vi "destroy function.vi"(11 "command in":string[](array[string])) -> ()   [LabVIEW 2011]
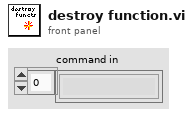
[diagram p1: front panel]
types:
  T1 = typedef "WPI_MotorControlDeviceRef.ctl" = cluster{"DeviceStatus":errorcluster, "Type":enum16{"PWM", "CAN"}, "PWM":cluster{"Digital Module":T2, "PWM Channel":T3, "DeadBand":T4}, "CAN":cluster{"Device Number":u8, "Control Mode":T5, "Semaphore":T6, "Max Vout":dbl}, "Invert":bool, "TransformRef":T7, "InvTransformRef":T7}
  T2 = typedef "FPGA_TypedefDigitalModule.ctl" = enum16{"Digital Module 1", "Digital Module 2"}
  T3 = typedef "FPGA_DIOPWMChannel.ctl" = enum8{"PWM 1", "PWM 2", "PWM 3", "PWM 4", "PWM 5", "PWM 6", "PWM 7", "PWM 8", "PWM 9", "PWM 10", "Invalid"}
  T4 = typedef "WPI_PWMDeadband.ctl" = cluster{"Name":string, "maxPositivePwm":i32, "minPositivePwm":i32, "centerPwm":i32, "maxNegativePwm":i32, "minNegativePwm":i32, "angularRange":u16}
  T5 = typedef "WPI_CANJaguar_ControlMode.ctl" = enum8{"Percent VBus", "Current", "Speed", "Position", "Voltage"}
  T6 = typedef "Semaphore RefNum" = refnum<k1>
  T7 = typedef "WPI_PWMTransform_ConPane.ctl" = refnum<vi>
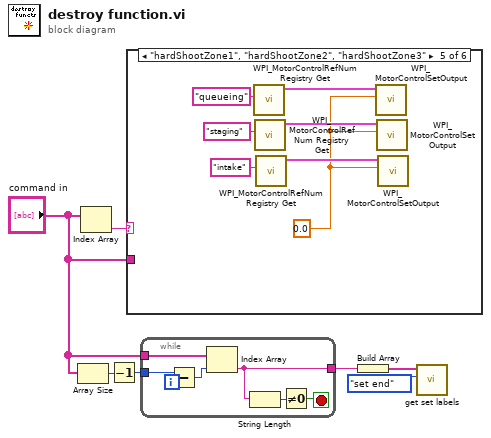
[diagram p0: block diagram]
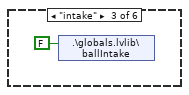
[diagram p4: hidden frame]
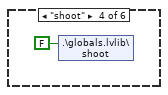
[diagram p5: hidden frame]
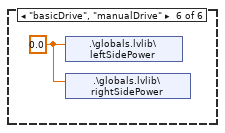
[diagram p6: hidden frame]
diagram:
  n1 = Array Size(array="command in") -> (size(s)=w6:i32)
  n2 = Index Array(array="command in") -> (element=w7:string)  [unwired: 1 in]
  n3 = Decrement(x=w6) -> (x-1=w5:i32)
  n4 = case shown="\"hardShootZone1\", \"hardShootZone2\", \"hardShootZone3\"" w7 {
    tunnel: "command in" -> [_ _ _ _ _ _]
    frame "testFunct" {
    }
    frame Default {
    }
    frame "intake" {
      n5 = shared-variable ".\\globals.lvlib\\ballIntake"(FALSE ("ballIntake")) -> ()  [unwired: 1 in, 1 out]
    }
    frame "shoot" {
      n6 = shared-variable ".\\globals.lvlib\\shoot"(FALSE ("shoot")) -> ()  [unwired: 1 in, 1 out]
    }
    frame "hardShootZone1", "hardShootZone2", "hardShootZone3" {
      w10 = 0.0 ("Output")
      n7 = call <vilib>:"WPI_MotorControlRefNum Registry Get.vi"("refnum name"="queueing") -> ("MotorControlDevRef"=w15:T1)  [unwired: 9 in, 1 out]
      n8 = call <vilib>:"WPI_MotorControlRefNum Registry Get.vi"("refnum name"="staging") -> ("MotorControlDevRef"=w14:T1)  [unwired: 9 in, 1 out]
      n9 = call <vilib>:"WPI_MotorControlRefNum Registry Get.vi"("refnum name"="intake") -> ("MotorControlDevRef"=w13:T1)  [unwired: 9 in, 1 out]
      n10 = call <vilib>:"WPI_MotorControlSetOutput.vi"("Output"=w10, "MotorControlDevRef"=w15) -> ()  [unwired: 8 in, 2 out]
      n11 = call <vilib>:"WPI_MotorControlSetOutput.vi"("Output"=w10, "MotorControlDevRef"=w14) -> ()  [unwired: 8 in, 2 out]
      n12 = call <vilib>:"WPI_MotorControlSetOutput.vi"("Output"=w10, "MotorControlDevRef"=w13) -> ()  [unwired: 8 in, 2 out]
    }
    frame "basicDrive", "manualDrive" {
      w17 = 0.0 ("Output")
      n13 = shared-variable ".\\globals.lvlib\\leftSidePower"(w17) -> ()  [unwired: 1 in, 1 out]
      n14 = shared-variable ".\\globals.lvlib\\rightSidePower"(w17) -> ()  [unwired: 1 in, 1 out]
    }
  }
  n15 = while {
    tunnel: "command in" -> [w22]
    tunnel: w5 -> [w23]
    tunnel: [w18] -> w2
    i -> [w24]
    stop <- w20 stop-if-true
    n16 = Subtract(x=w23, y=w24) -> (x-y=w21:i32)
    n17 = Index Array(array=w22, index=w21) -> (element=w18:string)
    n18 = String Length(string=w18) -> (length=w19:i32)
    n19 = Not Equal To 0?(x=w19) -> (x != 0?=w20:bool)
  }
  n20 = Build Array(w2) -> (w1:string[])
  n21 = call "get set labels.vi"("option in"=enum16{"get", "set", "remove", "set end"}."set end", "label in"=w1) -> ()  [unwired: 9 in, 1 out]
